vi "Establish_Var1.vi"(10 "SMU Config In":T1) -> (2 "Vname":string, 3 "SMU Config Out":T1)   [LabVIEW 2012]
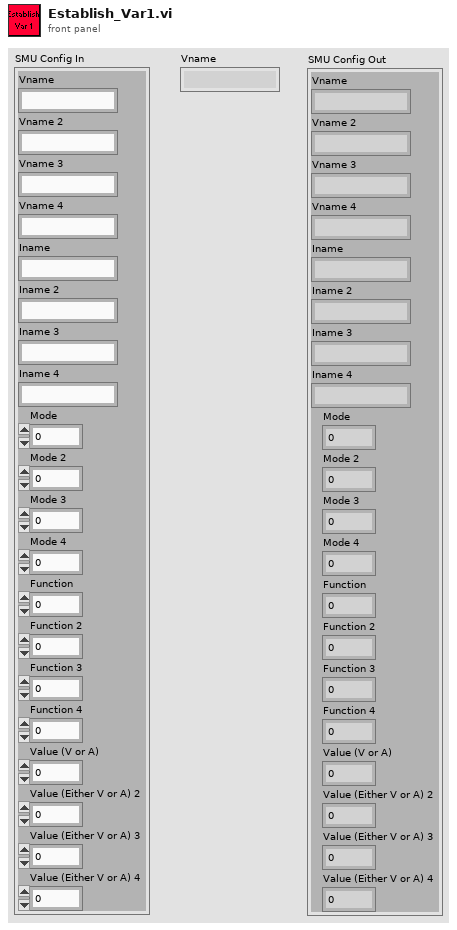
[diagram p1: front panel]
types:
  T1 = cluster{"Vname":string, "Vname 2":string, "Vname 3":string, "Vname 4":string, "Iname":string, "Iname 2":string, "Iname 3":string, "Iname 4":string, "Mode":u16, "Mode 2":u16, "Mode 3":u16, "Mode 4":u16, "Function":u16, "Function 2":u16, "Function 3":u16, "Function 4":u16, "Value (V or A)":dbl, "Value (Either V or A) 2":dbl, "Value (Either V or A) 3":dbl, "Value (Either V or A) 4":dbl}
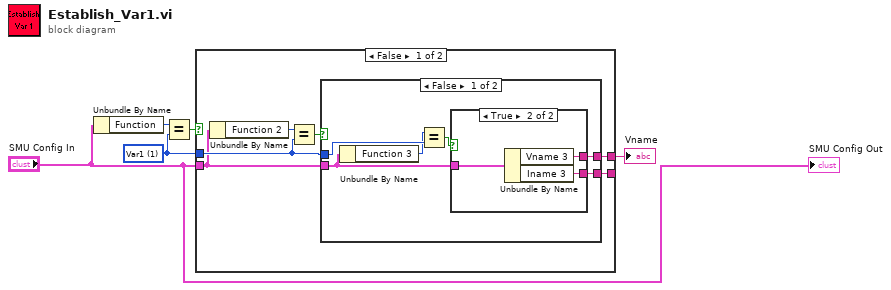
[diagram p0: block diagram]
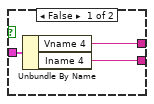
[diagram p2: hidden frame]
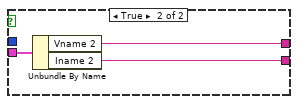
[diagram p3: hidden frame]
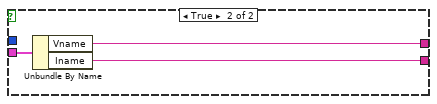
[diagram p4: hidden frame]
diagram:
  w3 = u16 1 items=["disabled", "Var1", "Var2", "Var1'", "Constant"] ("Function")
  n1 = Unbundle By Name("SMU Config In") -> ("Function"=w5:u16)
  n2 = Equal?(x=w5, y=w3) -> (x = y?=w2:bool)
  n3 = case shown="False" w2 {
    tunnel: [w10 w28] -> w4
    tunnel: [w11 w27] -> _
    tunnel: w3 -> [w8 _]
    tunnel: "SMU Config In" -> [w6 w29]
    frame False {
      n4 = Unbundle By Name(w6) -> ("Function 2"=w7:u16)
      n5 = Equal?(x=w7, y=w8) -> (x = y?=w9:bool)
      n6 = case shown="False" w9 {
        tunnel: [w14 w24] -> w11
        tunnel: [w15 w25] -> w10
        tunnel: w8 -> [w17 _]
        tunnel: w6 -> [w12 w26]
        frame False {
          n7 = Unbundle By Name(w12) -> ("Function 3"=w13:u16)
          n8 = Equal?(x=w13, y=w17) -> (x = y?=w16:bool)
          n9 = case shown="True" w16 {
            tunnel: [w19 w23] -> w15
            tunnel: [w18 w22] -> w14
            tunnel: w12 -> [w20 w21]
            frame False {
              n10 = Unbundle By Name(w20) -> ("Vname 4"=w19:string, "Iname 4"=w18:string)
            }
            frame True {
              n11 = Unbundle By Name(w21) -> ("Vname 3"=w23:string, "Iname 3"=w22:string)
            }
          }
        }
        frame True {
          n12 = Unbundle By Name(w26) -> ("Vname 2"=w25:string, "Iname 2"=w24:string)
        }
      }
    }
    frame True {
      n13 = Unbundle By Name(w29) -> ("Vname"=w28:string, "Iname"=w27:string)
    }
  }
  "Vname" <- w4
  "SMU Config Out" <- "SMU Config In"
